vi "Write Read after write.vi"(10 "Read after write":bool=TRUE, 11 "Device in":refnum<class "Device.lvclass">) -> (3 "Device out":refnum<class "Device.lvclass">)   [LabVIEW 2020, in "Device.lvclass"]
uses:
  Device.lvclass
  Device.lvclass/Device.ctl
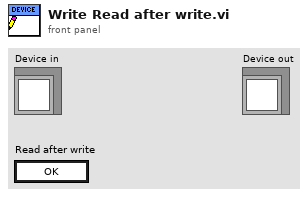
[diagram p1: front panel]
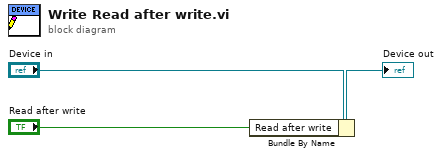
[diagram p0: block diagram]
diagram:
  n1 = Bundle By Name(cluster="Device in", "Read after write"="Read after write") -> (→"Device out":refnum<class "Device.lvclass">)
